vi "Get Trigger Level Range.vi"(10 "maximum":sgl, 11 "minimum":sgl) -> (1 "function return":u32, 2 "maximum out":sgl, 3 "minimum out":sgl)   [LabVIEW 2018, in "Copy of Andor SDK.lvlib"]
doc: "EXPNETTYPE unsigned int WINAPI GetTriggerLevelRange(float * minimum, float * maximum);"
uses:
  Copy of Andor SDK.lvlib
  <userlib>/Andor SDK/ATMCD32D.dll
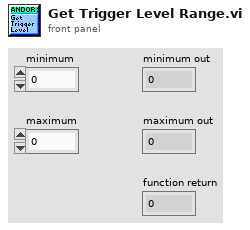
[diagram p1: front panel]
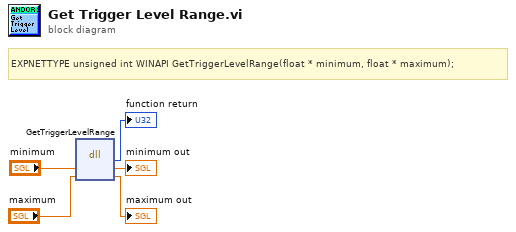
[diagram p0: block diagram]
diagram:
  # "EXPNETTYPE unsigned int WINAPI GetTriggerLevelRange(float * minimum, float * maximum);"
  n1 = dll-call lib="C:/Program Files (x86)/National Instruments/LabVIEW 2018/user.lib/Andor SDK/ATMCD32D.*" fn="GetTriggerLevelRange"("minimum"="minimum", "maximum"="maximum") -> (→"function return":u32, "minimum"=→"minimum out":sgl, "maximum"=→"maximum out":sgl)  [unwired: 3 in, 2 out]
